vi "Channel 0 Initiate Start Up (SubVI).vi"(10 "Channel # in":i32, 11 "VISA Refnum in":refnum<visa-resource-name>) -> (0 "error out":errorcluster, 1 "Channel # out":i32, 2 "BoardHandle out":T1, 3 "VISA Refnum out":refnum<visa-resource-name>)   [LabVIEW 2020]
uses:
  <instrlib>/CAEN PSM/CAEN PSM.lvlib
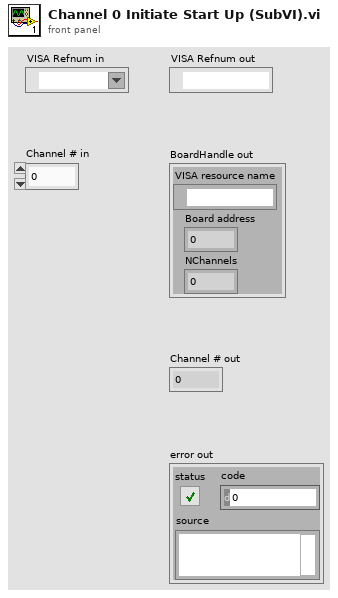
[diagram p1: front panel]
types:
  T1 = cluster{"VISA resource name":refnum<visa-resource-name>, "Board address":u8, "NChannels":u8}
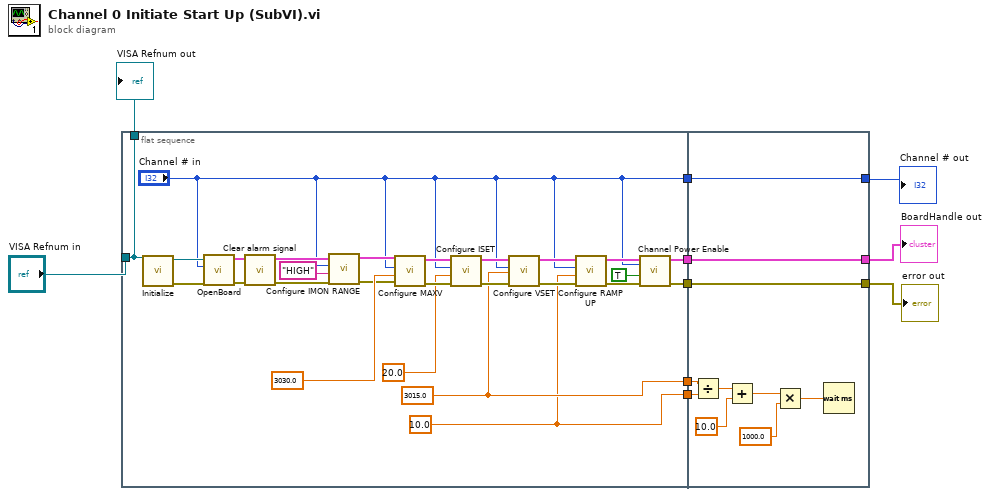
[diagram p0: block diagram]
diagram:
  n1 = flat-sequence {
    tunnel: [w22] -> w10
    tunnel: [w21] -> w9
    tunnel: [w18] -> w1
    tunnel: [w20] -> w8
    tunnel: [w19] -> w7
    tunnel: ["Channel # in"] -> w6
    tunnel: "VISA Refnum in" -> [w18]
    tunnel: w10 -> [w41]
    tunnel: w9 -> [w40]
    tunnel: [w39] -> w4
    tunnel: w8 -> [w39]
    tunnel: [w38] -> w3
    tunnel: w7 -> [w38]
    tunnel: [w37] -> w5
    tunnel: w6 -> [w37]
    frame #0 {
      w22 = 3015.0 ("Voltage Set (Volts)")
      w21 = 10.0 ("Voltage Ramp Up (V/s)")
      n2 = call <instrlib>:"Initialize.vi"("VISA resource name"=w18) -> ("error out"=w31:errorcluster, "VISA resource name out"=w28:refnum<visa-resource-name>)  [unwired: 9 in]
      n3 = call <instrlib>:"OpenBoard.vi"("error in (no error)"=w31, "Board Address"="Channel # in", "VISA resource name"=w28) -> ("error out"=w32:errorcluster, "BoardHandle"=w27:T1)  [unwired: 7 in]
      n4 = call <instrlib>:"Clear alarm signal.vi"("error in (no error)"=w32, "BoardHandle"=w27) -> ("error out"=w16:errorcluster, "BoardHandle out"=w15:T1)  [unwired: 8 in]
      n5 = call <instrlib>:"Configure IMON RANGE.vi"("error in (no error)"=w16, "IMon range (LOW)"="HIGH", "Channel (0)"="Channel # in", "BoardHandle"=w15) -> ("error out"=w12:errorcluster, "BoardHandle out"=w13:T1)  [unwired: 6 in]
      n6 = call <instrlib>:"Configure MAXV.vi"("error in (no error)"=w12, "Voltage Max (0.0 V)"=3030.0 ("VMax (Volts)"), "Channel (0)"="Channel # in", "BoardHandle"=w13) -> ("error out"=w33:errorcluster, "BoardHandle out"=w26:T1)  [unwired: 6 in]
      n7 = call <instrlib>:"Configure ISET.vi"("error in (no error)"=w33, "Current Limit (0.00 uA)"=20.0 ("Current Limit (uA)"), "Channel (0)"="Channel # in", "BoardHandle"=w26) -> ("error out"=w34:errorcluster, "BoardHandle out"=w25:T1)  [unwired: 6 in]
      n8 = call <instrlib>:"Configure VSET.vi"("error in (no error)"=w34, "Voltage Level (0.0 V)"=w22, "Channel (0)"="Channel # in", "BoardHandle"=w25) -> ("error out"=w35:errorcluster, "BoardHandle out"=w24:T1)  [unwired: 6 in]
      n9 = call <instrlib>:"Configure RAMP UP.vi"("error in (no error)"=w35, "Voltage ramp up (0 V/s)"=w21, "Channel (0)"="Channel # in", "BoardHandle"=w24) -> ("error out"=w36:errorcluster, "BoardHandle out"=w23:T1)  [unwired: 6 in]
      n10 = call <instrlib>:"Channel Power Enable.vi"("error in (no error)"=w36, "Enable (OFF)"=TRUE ("Boolean"), "Channel (0)"="Channel # in", "BoardHandle"=w23) -> ("error out"=w19:errorcluster, "BoardHandle out"=w20:T1)  [unwired: 6 in]
    }
    frame #1 {
      n11 = Divide(x=w41, y=w40) -> (x/y=w44:dbl)
      n12 = Add(x=w44, y=10.0) -> (x+y=w45:dbl)
      n13 = Multiply(x=w45, y=1000.0) -> (x*y=w46:dbl)
      n14 = Wait (ms)(milliseconds to wait=w46) -> ()  [unwired: 1 out]
    }
  }
  "Channel # out" <- w5
  "BoardHandle out" <- w4
  "error out" <- w3
  "VISA Refnum out" <- w1
